vi "Find Item in Library.vi"(7 "Item Type":string, 8 "error in (no error)":errorcluster, 10 "Item Name":string, 11 "Library item in":refnum<vi>) -> (0 "error out":errorcluster, 1 "Found?":bool, 2 "Project Item (Library Item)":refnum<vi>, 3 "Library item out":refnum<vi>)   [LabVIEW 2019, in "gRPC Template Creation Utility.lvlib"]
uses:
  gRPC Template Creation Utility.lvlib
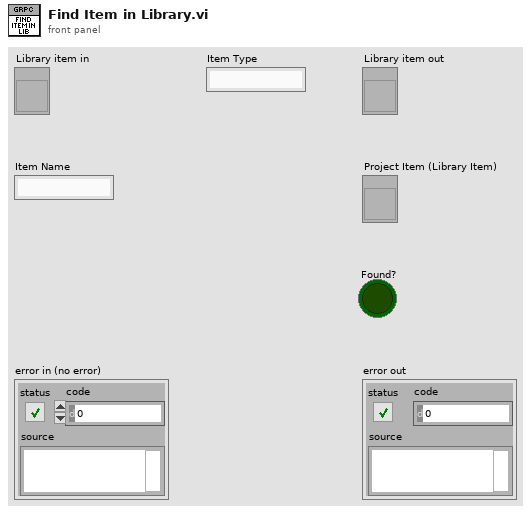
[diagram p1: front panel]
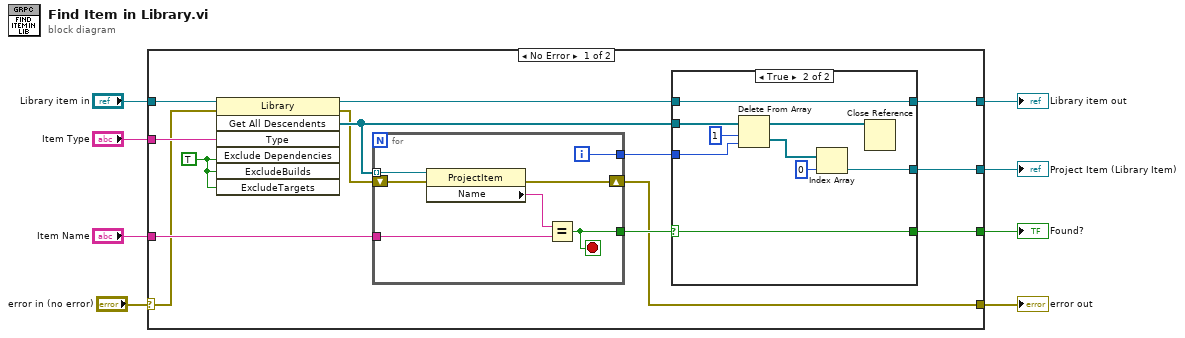
[diagram p0: block diagram]
diagram:
  n1 = case shown="No Error" "error in (no error)" {
    selector: "error in (no error)" -> [w16 w41]
    tunnel: "Item Name" -> [w22 _]
    tunnel: "Item Type" -> [w18 _]
    tunnel: "Library item in" -> [w17 w42]
    tunnel: [w11 w42] -> w2
    tunnel: [w13 _] -> w4
    tunnel: [w15 _] -> w3
    tunnel: [w9 w41] -> w1
    frame No Error {
      w19 = TRUE ("ExcludeDependencies")
      n2 = invoke class="Library" method="Get All Descendents"(reference=w17, error in=w16, "Type"=w18, "Exclude Dependencies"=w19, "ExcludeBuilds"=w19, "ExcludeTargets"=w19) -> (reference out=w12:refnum<vi>, error out=w10:errorcluster, "All Descendents"=w20:refnum<vi>[])  [unwired: 1 in, 4 out]
      n3 = for {
        tunnel: w20 -> [w40] mode=indexing
        tunnel: [w38] -> w21
        tunnel: [w37] -> w14
        tunnel: w22 -> [w36]
        shift-right: [w34] -> w9
        shift-left: w10 -> [w35]
        i -> [w38]
        stop <- w37 stop-if-true
        n4 = property class="ProjectItem"(reference=w40, error in=w35) -> (error out=w34:errorcluster, "Name"=w39:string)  [unwired: 1 out]
        n5 = Equal?(x=w39, y=w36) -> (x = y?=w37:bool)
      }
      n6 = case shown="True" w14 {
        selector: w14 -> [w23 w26]
        tunnel: w21 -> [_ w31]
        tunnel: w20 -> [_ w30]
        tunnel: [_ w27] -> w15
        tunnel: [w23 w26] -> w13
        tunnel: w12 -> [w24 w25]
        tunnel: [w24 w25] -> w11
        frame False {
        }
        frame True {
          n7 = Delete From Array(array=w30, length=1, index=w31) -> (deleted portion=w29:refnum<vi>[], array with subset deleted=w33:refnum<vi>[])
          n8 = Index Array(array=w29, index=0) -> (element=w27:refnum<vi>)
          n9 = Close Reference(reference=w33) -> ()  [unwired: 1 in, 1 out]
        }
      }
    }
    frame Error {
    }
  }
  "Project Item (Library Item)" <- w3
  "Found?" <- w4
  "Library item out" <- w2
  "error out" <- w1
